vi "Elevator_Teleop.vi"(0 "Joystick_Out":T1, 1 "Visited_Disabled":bool) -> ()   [LabVIEW 2018]
uses:
  Utility_VIs/Joystick_Controls.ctl
  Subsytems/Elevator/Elevator_Notifier.ctl
  Subsytems/Elevator/Elevator_Control_Type.ctl
  Subsytems/Elevator/Elevator_Enum_States.ctl
  Global_Variables/Elevator_Globals.vi
  Global_Variables/Climb_Globals.vi
  Global_Variables/Sensor_Values.vi
panel:
  out "Climb_Advance Elevator":bool
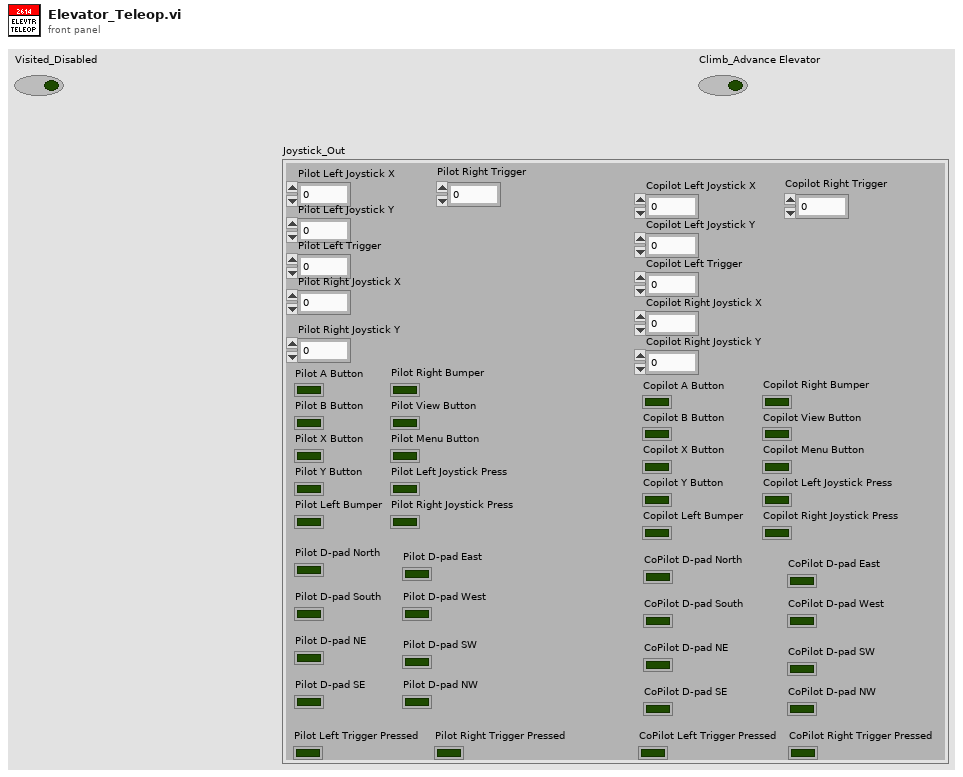
[diagram p1: front panel]
types:
  T1 = typedef "Joystick_Controls.ctl" = cluster{"Pilot Left Joystick X":dbl, "Pilot Left Joystick Y":dbl, "Pilot A Button":bool, "Pilot B Button":bool, "Pilot X Button":bool, "Pilot Y Button":bool, "Pilot Left Bumper":bool, "Pilot Right Bumper":bool, "Pilot View Button":bool, "Pilot Menu Button":bool, "Pilot Left Joystick Press":bool, "Pilot Right Joystick Press":bool, "Pilot Left Trigger":dbl, "Pilot Right Joystick X":dbl, "Pilot Right Joystick Y":dbl, "Pilot Right Trigger":dbl, "Copilot Left Joystick X":dbl, "Copilot Left Joystick Y":dbl, "Copilot A Button":bool, "Copilot B Button":bool, "Copilot X Button":bool, "Copilot Y Button":bool, "Copilot Left Bumper":bool, "Copilot Right Bumper":bool, "Copilot View Button":bool, "Copilot Menu Button":bool, "Copilot Left Joystick Press":bool, "Copilot Right Joystick Press":bool, "Copilot Left Trigger":dbl, "Copilot Right Joystick X":dbl, "Copilot Right Joystick Y":dbl, "Copilot Right Trigger":dbl, "Pilot D-pad North":bool, "Pilot D-pad South":bool, "Pilot D-pad East":bool, "Pilot D-pad West":bool, "Pilot D-pad NE ":bool, "Pilot D-pad SE":bool, "Pilot D-pad SW":bool, "Pilot D-pad NW":bool, "CoPilot D-pad North":bool, "CoPilot D-pad South":bool, "CoPilot D-pad East":bool, "CoPilot D-pad West":bool, "CoPilot D-pad NE":bool, "CoPilot D-pad SE":bool, "CoPilot D-pad SW":bool, "CoPilot D-pad NW":bool, "Pilot Left Trigger Pressed":bool, "Pilot Right Trigger Pressed":bool, "CoPilot Left Trigger Pressed":bool, "CoPilot Right Trigger Pressed":bool}
  T2 = typedef "Elevator_Notifier.ctl" = cluster{"Elevator_Control_Type":T3, "Shift":bool, "Brake":bool, "Manual_Lift_Up":bool, "Manual_Lift_Down":bool, "Climb_Advance":bool, "Climb_Reverse":bool, "Low_Rocket":bool, "Mid_Rocket":bool, "High_Rocket":bool, "Cargo_Ship":bool, "Hatch_Floor":bool, "Cargo_Floor":bool, "HP_Hatch":bool, "HP_Cargo":bool, "Depot_Cargo":bool, "Stow":bool, "Set_Position":T4, "Intake_Mode":bool, "Climb_Distance":dbl, "Level_Two":bool, "Parameter_One":dbl, "Parameter_Two":dbl, "Parameter_Three":dbl, "Step":i32, "Elevator_Notifier":refnum<notifier>, "Brake_State":bool, "Shift_State":bool}
  T3 = typedef "Elevator_Control_Type.ctl" = enum16{"No_Op", "Shift", "Brake", "Manual_Elevator_Up", "Manual_Elevator_Down", "Manual_Climb_Up", "Manual_Climb_Down", "Manual_Position_Control", "Elevator_Retract", "Elevator_Extend", "Brake_In_Climb", "Position_Control", "Position", "Shift_Climb"}
  T4 = typedef "Elevator_Enum_States.ctl" = enum16{"Current_Position", "High_Rocket_Hatch_Panel_Floor", "High_Rocket_Hatch_Panel", "Mid_Rocket_Hatch_Panel_Floor", "Mid_Rocket_Hatch_Panel", "Low_Rocket_Hatch_Panel", "Cargo_Ship_Hatch_Panel", "Loading_Station_Hatch_Panel", "Ground_Pickup_Hatch_Panel", "High_Rocket_Cargo", "Mid_Rocket_Cargo", "Low_Rocket_Cargo", "Cargo_Ship_Cargo", "Loading_Station_Cargo", "Ground_Pickup_Cargo", "Depot_Pickup_Cargo", "Descend_Off_Platform", "Stow_Cargo"}
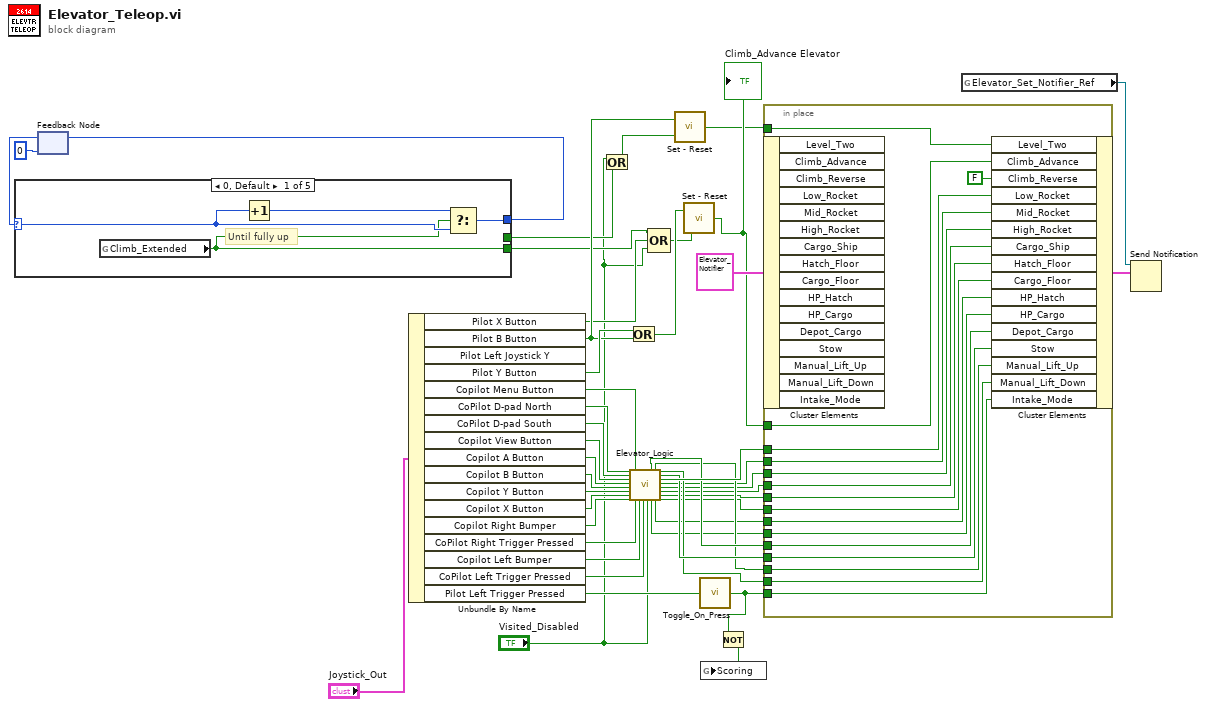
[diagram p0: block diagram]
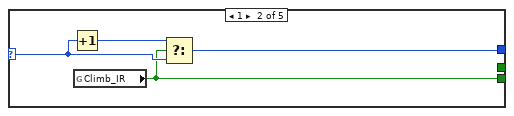
[diagram p2: hidden frame]
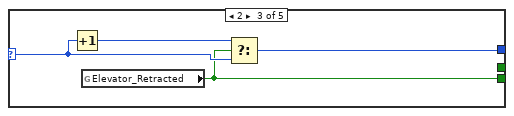
[diagram p3: hidden frame]
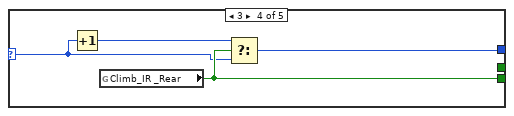
[diagram p4: hidden frame]
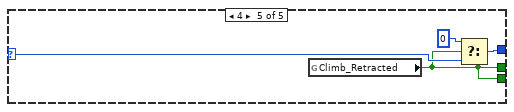
[diagram p5: hidden frame]
diagram:
  n1 = feedback #1(0) -> (w10:i32)
  n2 = case shown="0, Default" w10 {
    selector: w10 -> [w48 w51 w55 w59 w64]
    tunnel: [w47 w53 w56 w61 w65] -> w9
    tunnel: [w46 w50 w54 w60 w62] -> w4
    tunnel: [_ _ _ _ w62] -> w6
    frame 0, Default {
      # "Until fully up"
      n3 = global read "Climb_Globals.vi" "Climb_Extended"() -> (w46:bool)
      n4 = Increment(x=w48) -> (x+1=w49:i32)
      n5 = Select(t=w49, s=w46, f=w48) -> (s? t:f=w47:i32)
    }
    frame 1 {
      n6 = Increment(x=w51) -> (x+1=w52:i32)
      n7 = global read "Sensor_Values.vi" "Climb_IR"() -> (w50:bool)
      n8 = Select(t=w52, s=w50, f=w51) -> (s? t:f=w53:i32)
    }
    frame 2 {
      n9 = Increment(x=w55) -> (x+1=w57:i32)
      n10 = global read "Elevator_Globals.vi" "Elevator_Retracted"() -> (w54:bool)
      n11 = Select(t=w57, s=w54, f=w55) -> (s? t:f=w56:i32)
    }
    frame 3 {
      n12 = Increment(x=w59) -> (x+1=w58:i32)
      n13 = global read "Sensor_Values.vi" "Climb_IR _Rear"() -> (w60:bool)
      n14 = Select(t=w58, s=w60, f=w59) -> (s? t:f=w61:i32)
    }
    frame 4 {
      n15 = global read "Climb_Globals.vi" "Climb_Retracted"() -> (w62:bool)
      n16 = Select(t=0, s=w62, f=w64) -> (s? t:f=w65:i32)
    }
  }
  n17 = feedback-in #1(w9) -> ()
  n18 = Unbundle By Name("Joystick_Out") -> ("Pilot X Button"=w3:bool, "Pilot B Button"=w7:bool, "Pilot Y Button"=w41:bool, "Copilot Menu Button"=w28:bool, "CoPilot D-pad North"=w27:bool, "CoPilot D-pad South"=w26:bool, "Copilot View Button"=w25:bool, "Copilot A Button"=w24:bool, "Copilot B Button"=w23:bool, "Copilot Y Button"=w22:bool, "Copilot X Button"=w21:bool, "Copilot Right Bumper"=w20:bool, "CoPilot Right Trigger Pressed"=w19:bool, "Copilot Left Bumper"=w18:bool, "CoPilot Left Trigger Pressed"=w17:bool, "Pilot Left Trigger Pressed"=w16:bool)  [unwired: 1 out]
  n19 = Or(x="Visited_Disabled", y=w6) -> (x .or. y?=w2:bool)
  n20 = Or(x=w41, y=w7) -> (x .or. y?=w12:bool)
  n21 = call "Elevator_Logic.vi"("Manual_Up"=w27, "Manual_Down"=w26, "Stow"=w25, "Low_Rocket"=w24, "Mid_Rocket"=w23, "High_Rocket"=w22, "Cargo_Ship"=w21, "Hatch_Floor"=w20, "Depot_Cargo"=w28, "Cargo_Floor"=w19, "HP_Hatch"=w18, "HP_Cargo"=w17, "Visited_Disabled"="Visited_Disabled") -> ("Depot_Cargo_Out"=w38:bool, "HP_Cargo_Out"=w29:bool, "Manual_Up_Out"=w37:bool, "HP_Hatch_Out"=w30:bool, "Manual_Down_Out"=w36:bool, "Stow_Out"=w39:bool, "Low_Rocket_Out"=w40:bool, "Mid_Rocket_Out"=w35:bool, "High_Rocket_Out"=w34:bool, "Cargo_Ship_Out"=w33:bool, "Hatch_Floor_Out"=w32:bool, "Cargo_Floor_Out"=w31:bool)  [unwired: 3 in]
  n22 = Compound Arithmetic op=OR(w4, w3, "Visited_Disabled") -> (w5:bool)
  n23 = call "Set - Reset.vi"("Reset"=w2, "Set"=w7) -> ("Output"=w8:bool)
  n24 = call "Set - Reset.vi"("Reset"=w5, "Set"=w12) -> ("Output"=w13:bool)
  "Climb_Advance Elevator" <- w13
  n25 = call "Toggle_On_Press.vi"("Boolean"=w16) -> ("Boolean Out"=w15:bool)
  n26 = Not(x=w15) -> (.not. x?=w14:bool)
  n27 = global write "Elevator_Globals.vi" "Scoring"(w14) -> ()
  n28 = in-place {
    in-place-border: w13 -> [w81]
    in-place-border: w40 -> [w80]
    in-place-border: w39 -> [w79]
    in-place-border: w38 -> [w78]
    in-place-border: w37 -> [w77]
    in-place-border: w36 -> [w76]
    in-place-border: w35 -> [w75]
    in-place-border: w34 -> [w74]
    in-place-border: w33 -> [w73]
    in-place-border: w32 -> [w72]
    in-place-border: w31 -> [w71]
    in-place-border: w30 -> [w70]
    in-place-border: w29 -> [w69]
    in-place-border: w15 -> [w68]
    in-place-border: w8 -> [w67]
    n29 = in-place-cluster #2(T2 {"Elevator_Control_Type"=enum."No_Op", "Shift"=FALSE, "Brake"=FALSE, "Manual_Lift_Up"=FALSE, "Manual_Lift_Down"=FALSE, "Climb_Advance"=FALSE, "Climb_Reverse"=FALSE, "Low_Rocket"=FALSE, "Mid_Rocket"=FALSE, "High_Rocket"=FALSE, "Cargo_Ship"=FALSE, "Hatch_Floor"=FALSE, "Cargo_Floor"=FALSE, "HP_Hatch"=FALSE, "HP_Cargo"=FALSE, "Depot_Cargo"=FALSE, "Stow"=FALSE, "Set_Position"=enum."High_Rocket_Hatch_Panel", "Intake_Mode"=FALSE, "Climb_Distance"=0.0, "Level_Two"=FALSE, "Parameter_One"=0.0, "Parameter_Two"=0.0, "Parameter_Three"=0.0, "Step"=0, "Elevator_Notifier"=refnum, "Brake_State"=FALSE, "Shift_State"=FALSE} ("Elevator_Notifier")) -> ()  [unwired: 16 out]
    n30 = in-place-cluster #2("Level_Two"=w67, "Climb_Advance"=w81, "Climb_Reverse"=FALSE, "Low_Rocket"=w80, "Mid_Rocket"=w75, "High_Rocket"=w74, "Cargo_Ship"=w73, "Hatch_Floor"=w72, "Cargo_Floor"=w71, "HP_Hatch"=w70, "HP_Cargo"=w69, "Depot_Cargo"=w78, "Stow"=w79, "Manual_Lift_Up"=w77, "Manual_Lift_Down"=w76, "Intake_Mode"=w68) -> (w45:T2)
  }
  n31 = global read "Elevator_Globals.vi" "Elevator_Set_Notifier_Ref"() -> (w44:refnum<notifier>)
  n32 = Send Notification(notification=w45, notifier=w44) -> ()  [unwired: 1 in, 2 out]
